vi "version_read.vi"(8 "error in (no error)":errorcluster, 11 "lv-build in":refnum<class "lv-builder-default.lvclass">) -> (0 "error out":errorcluster, 2 "version":string, 3 "lv-build out":refnum<class "lv-builder-default.lvclass">)   [LabVIEW 2015, in "lv-builder-default.lvclass"]
uses:
  lv-builder-default.lvclass
  lv-builder-default.lvclass/lv-builder-default.ctl
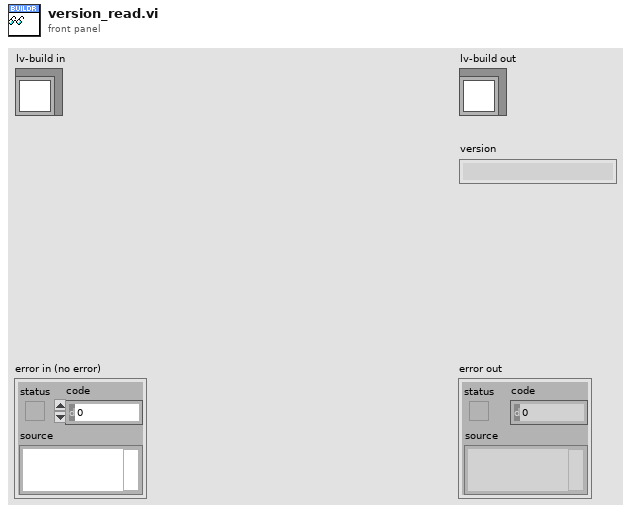
[diagram p1: front panel]
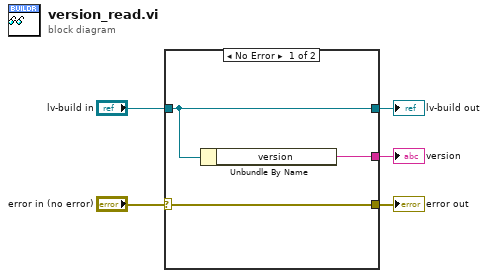
[diagram p0: block diagram]
diagram:
  n1 = case shown="No Error" "error in (no error)" {
    selector: "error in (no error)" -> [w8 w10]
    tunnel: [w8 w10] -> w4
    tunnel: "lv-build in" -> [w6 w9]
    tunnel: [w6 w9] -> w2
    tunnel: [w7 _] -> w1
    frame No Error {
      n2 = Unbundle By Name(w6) -> ("version"=w7:string)
    }
    frame Error {
    }
  }
  "error out" <- w4
  "lv-build out" <- w2
  "version" <- w1
